vi "_Set Oscillator.vi"   [LabVIEW 2012]
uses:
  Type/_FPGA Chip Type.ctl
  <vilib>/rvi/DataTransferAndStorage/Container/Common/niFpgaContainerGetUniqueNameForEmu.vi
  <vilib>/rvi/Memory/Memory_Emulation/niFpgaMemoryEmulationCacheClearOnFirstRun.vi
  <vilib>/rvi/Memory/Memory_Emulation/nirvimemoryEmulationManagerCache_MakeExclusive.vi
  <vilib>/rvi/Memory/Memory_Emulation/niFpgaMemoryEmulationValidateCache.vi
  <vilib>/rvi/Memory/Memory_Emulation/nirvimemoryEmulationManagerCache_ReleaseExclusive.vi
  <vilib>/rvi/Memory/Memory_Emulation/nirvimemoryEmulationManagerCache_InsertValue.vi
  <vilib>/Utility/error.llb/Clear Errors.vi
  <vilib>/rvi/Memory/Memory_Emulation/nirvimemoryEmulationManagerCache_GetValue.vi
  <vilib>/rvi/DataTransferAndStorage/Container/XNode/niFpgaContainer.xnode
  <vilib>/rvi/Memory/Memory_Emulation/nirvimemoryEmulation.vi
types:
  T1 = typedef "_FPGA Chip Type.ctl" = enum8{"None", "ADC1", "ADC2", "ADC3", "ADC4", "ADC5", "ADC6", "ADC7", "ADC8", "ADC9", "ADC10", "ADC11", "ADC12", "ADC13", "DAC1", "DAC2", "DAC3", "DAC4", "DAC5", "LENS1", "LENS2", "LENS3", "LENS4", "LENS5", "LENS6", "LENS7", "MASS1", "MASS2", "MASS3", "MASS4", "MASS5", "OSC1", "OSC2", "OSC3", "LATCH1", "LATCH2", "LATCH3", "LATCH4", "PIC1", "PIC2", "PIC3", "PIC4"}
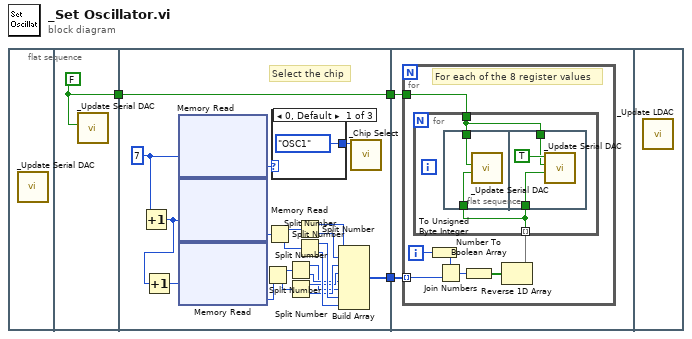
[diagram p0: block diagram]
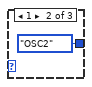
[diagram p2: hidden frame]
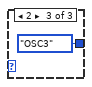
[diagram p3: hidden frame]
diagram:
  n1 = flat-sequence {
    tunnel: [w4] -> w1
    tunnel: [w17] -> w3
    tunnel: [w5] -> w2
    tunnel: w1 -> [w5]
    tunnel: w3 -> [w30]
    tunnel: w2 -> [w29]
    frame #0 {
      n2 = call "_Update Serial DAC.vi"() -> ()  [unwired: 4 in, 4 out]
    }
    frame #1 {
      w4 = FALSE
      n3 = call "_Update Serial DAC.vi"("FSYNCH (T)"=w4) -> ()  [unwired: 3 in, 4 out]
    }
    frame #2 {
      w8 = u8 7 ("Address")
      # "Select the chip"
      n4 = Increment(x=w8) -> (x+1=w7:u8)
      n5 = Increment(x=w7) -> (x+1=w9:u8)
      n6 = xnode ("Memory Read")("Address"=w8) -> ("Data"=w6:u32)  [unwired: 1 in, 1 out]
      n7 = xnode ("Memory Read")("Address"=w7) -> ("Data"=w16:u32)  [unwired: 1 in, 1 out]
      n8 = xnode ("Memory Read")("Address"=w9) -> ("Data"=w15:u32)  [unwired: 1 in, 1 out]
      n9 = Split Number(x=w15) -> (hi(x)=w22:u16, lo(x)=w23:u16)
      n10 = Split Number(x=w16) -> (hi(x)=w25:u16, lo(x)=w24:u16)
      n11 = case shown="0, Default" w6 {
        tunnel: [_FPGA_Chip_Type."OSC1" ("ChipType") _FPGA_Chip_Type."OSC2" ("ChipType") _FPGA_Chip_Type."OSC3" ("ChipType")] -> w14
        frame 0, Default {
        }
        frame 1 {
        }
        frame 2 {
        }
      }
      n12 = Split Number(x=w22) -> (hi(x)=w10:u8, lo(x)=w11:u8)
      n13 = Split Number(x=w23) -> (hi(x)=w12:u8, lo(x)=w13:u8)
      n14 = Split Number(x=w25) -> (hi(x)=w21:u8, lo(x)=w20:u8)
      n15 = Split Number(x=w24) -> (hi(x)=w19:u8, lo(x)=w18:u8)
      n16 = Build Array(w21, w20, w13, w12, w11, w10, w19, w18) -> (w17:u8[])
      n17 = call "_Chip Select.vi"("ChipType"=w14) -> ()  [unwired: 1 in, 6 out]
    }
    frame #3 {
      n18 = for {
        tunnel: w30 -> [w33] mode=indexing
        tunnel: w29 -> [w31]
        i -> [w37]
        # "For each of the 8 register values"
        n19 = To Unsigned Byte Integer(number=w37) -> (unsigned 8bit integer=w32:u8)
        n20 = Join Numbers(hi=w32, lo=w33) -> ((hi.lo)=w34:u16)
        n21 = Number To Boolean Array(number=w34) -> (Boolean array=w36:bool[])
        n22 = Reverse 1D Array(array=w36) -> (reversed array=w35:bool[])
        n23 = for {
          tunnel: w35 -> [w39] mode=indexing
          tunnel: w31 -> [w38]
          n24 = flat-sequence {
            tunnel: w39 -> [w41]
            tunnel: w38 -> [w40]
            tunnel: w39 -> [w44]
            tunnel: w38 -> [w42]
            frame #0 {
              n25 = call "_Update Serial DAC.vi"("DIN (F)"=w41, "FSYNCH (T)"=w40) -> ()  [unwired: 2 in, 4 out]
            }
            frame #1 {
              n26 = call "_Update Serial DAC.vi"("DIN (F)"=w44, "FSYNCH (T)"=w42, "Clock (F)"=TRUE ("Clock")) -> ()  [unwired: 1 in, 4 out]
            }
          }
        }
      }
    }
    frame #4 {
      n27 = call "_Update LDAC.vi"() -> ()  [unwired: 6 out]
    }
  }
